vi "Tol_Check.vi"(8 "Lower Error Bound":dbl, 9 "Upper Error Bound":dbl, 10 "Process Variable":dbl, 11 "Setpoint":dbl) -> (3 "In Range?":bool)   [LabVIEW 2016]
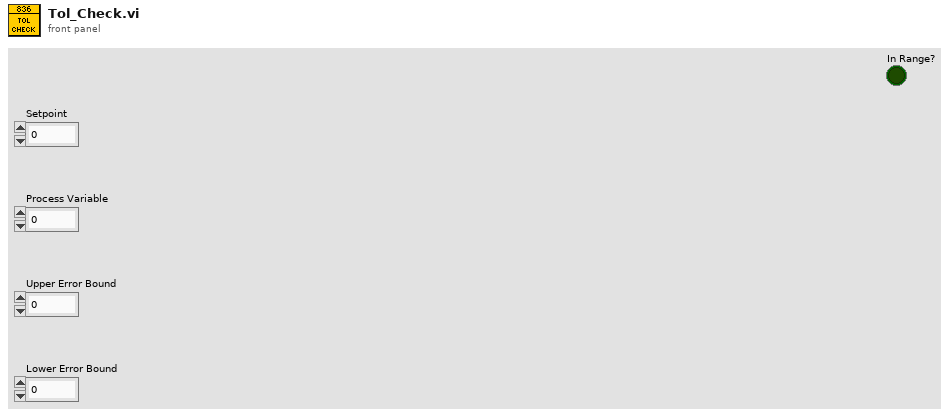
[diagram p1: front panel]
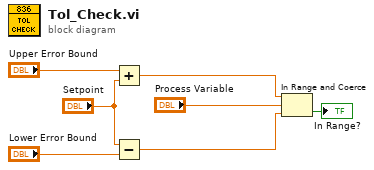
[diagram p0: block diagram]
diagram:
  n1 = Add(x="Upper Error Bound", y="Setpoint") -> (x+y=w4:dbl)
  n2 = Subtract(x="Setpoint", y="Lower Error Bound") -> (x-y=w3:dbl)
  n3 = In Range and Coerce(upper limit=w4, x="Process Variable", lower limit=w3) -> (In Range?=→"In Range?":bool)  [unwired: 1 out]
